vi "Test Suite from Project.vi"(8 "error in (no error)":errorcluster, 11 "Test Case In":refnum<class "LUnit Test Suite Tests.lvclass">) -> (0 "error out":errorcluster, 3 "Test Case Out":refnum<class "LUnit Test Suite Tests.lvclass">)   [LabVIEW 2020, in "LUnit Test Suite Tests.lvclass"]
uses:
  LUnit Test Suite Tests.lvclass
  LUnit Test Suite Tests.lvclass/LUnit Test Suite Tests.ctl
  source/Framework/Test Finder/Test Finder.lvclass
  Test Doubles/Test Case Test Double Child/Light Test Case Double.lvclass
  C:/git/astemes-lunit/source/LUnit Test Case.lvclass
  C:/git/astemes-lunit/source/Runnable.lvclass
  C:/git/astemes-lunit/tests/Test Doubles/Test Case Test Double Child/Light Test Case Double.lvclass
  source/LUnit Test Suite.lvclass
  C:/git/astemes-lunit/source/LUnit Test Suite.lvclass
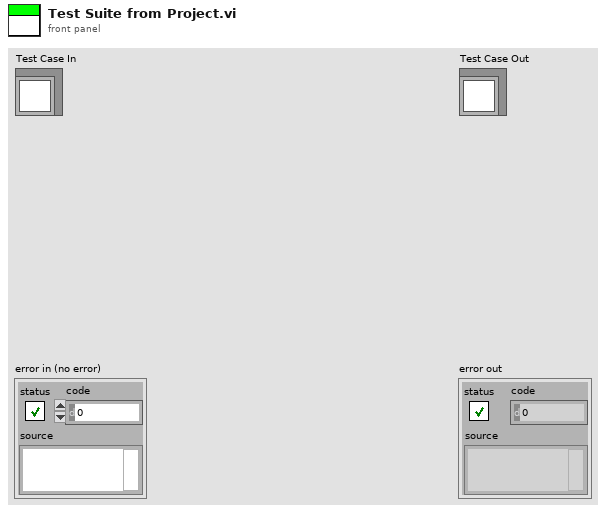
[diagram p1: front panel]
types:
  T1 = typedef "Result.lvlib/Result.ctl" = cluster{"Name":string, "Description":string, "Status":T2, "Result Type":T3, "Execution Time":dbl, "Data":cluster{"Expected":variant, "Actual":variant, "Delta":variant}}
  T2 = typedef "Result.lvlib/Status.ctl" = enum16{"", "Passed", "Failed", "Error", "Skipped", "Setup Error", "Broken", "Teardown Error"}
  T3 = typedef "Result.lvlib/Type.ctl" = enum16{"Test Case", "Test Suite", "Test Run", "Pass", "Fail", "Skip", "Pass if", "Fail if", "Pass if Error", "Fail if Error", "Pass if Equal", "Fail if Equal"}
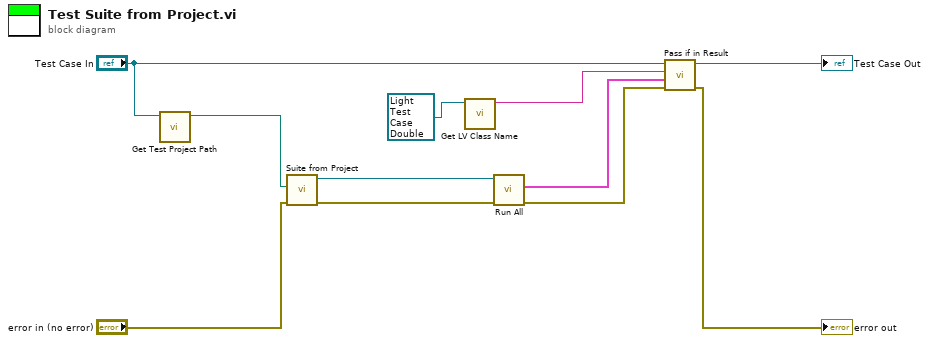
[diagram p0: block diagram]
diagram:
  n1 = call "Get Test Project Path.vi"("LUnit Test Suite Tests in"="Test Case In") -> ("appended path"=w2:path)  [unwired: 10 in]
  n2 = call "Suite from Project.vi"("error in (no error)"="error in (no error)", "Project Path"=w2) -> ("error out"=w7:errorcluster, "LUnit Test Suite Out"=w8:refnum<class "LUnit Test Suite.lvclass">)  [unwired: 8 in]
  n3 = call <vilib>:"Get LV Class Name.vi"("object"=refnum<class "Light Test Case Double.lvclass"> refnum ("Light Test Case Double.lvclass")) -> ("class name"=w3:string)  [unwired: 9 in, 1 out]
  n4 = call "Run All.vi"("error in (no error)"=w7, "Runnable In"=w8) -> ("error out"=w6:errorcluster, "Results"=w1:T1[])  [unwired: 8 in]
  n5 = call "Pass if in Result.vi"("error in (no error)"=w6, "Results"=w1, "Method Name"=w3, "LUnit Test Suite Tests in"="Test Case In") -> ("error out"=→"error out":errorcluster, "LUnit Test Suite Tests out"=→"Test Case Out":refnum<class "LUnit Test Suite Tests.lvclass">)  [unwired: 6 in]
